vi "FindPrjLibItem.vi"(8 "error in (no error)":errorcluster, 10 "Item Name":string, 11 "Lib Path":path) -> (0 "error out":errorcluster, 3 "ProjectItem Refnum":refnum<vi>)   [LabVIEW 2020, in "CameraI2COUSB.lvlib" / "CameraDemo.lvclass"]
uses:
  CameraDemo.lvclass
  CameraDemo.lvclass/CameraDemo.ctl
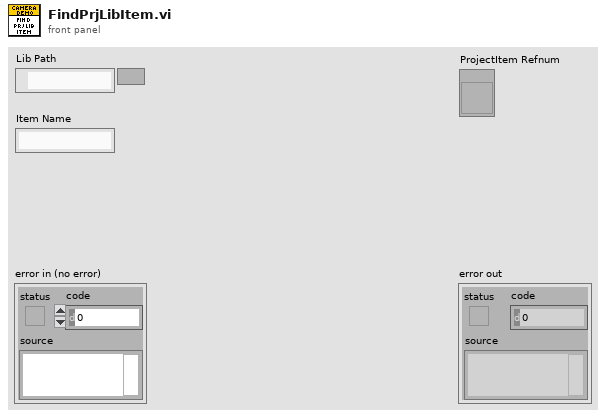
[diagram p1: front panel]
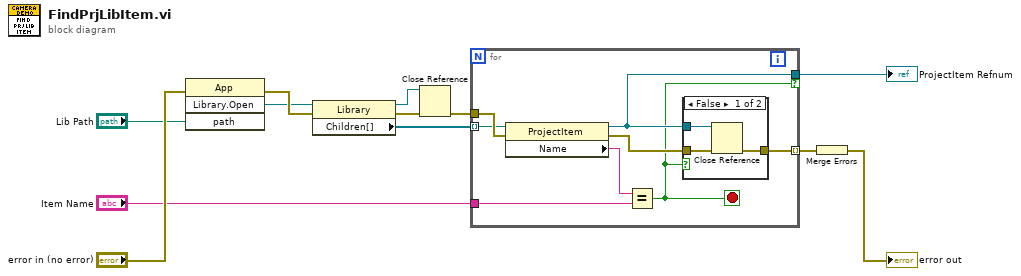
[diagram p0: block diagram]
diagram:
  n1 = invoke class="App" method="Library.Open"(error in="error in (no error)", "path"="Lib Path") -> (error out=w12:errorcluster, "Open Library"=w11:refnum<vi>)  [unwired: 2 in, 2 out]
  n2 = property class="Library"(reference=w11, error in=w12) -> (reference out=w9:refnum<vi>, error out=w10:errorcluster, "Children[]"=w7:refnum<vi>[])
  n3 = Close Reference(reference=w9, error in (no error)=w10) -> (error out=w8:errorcluster)
  n4 = for {
    tunnel: w7 -> [w16] mode=indexing
    tunnel: w8 -> [w19]
    tunnel: [w15] -> w3 mode=indexing
    tunnel: "Item Name" -> [w18]
    tunnel: [w14] -> w1 if=w13
    stop <- w13 stop-if-true
    n5 = property class="ProjectItem"(reference=w16, error in=w19) -> (reference out=w14:refnum<vi>, error out=w17:errorcluster, "Name"=w20:string)
    n6 = Equal?(x=w20, y=w18) -> (x = y?=w13:bool)
    n7 = case shown="False" w13 {
      tunnel: w17 -> [w23 w24]
      tunnel: w14 -> [w21 _]
      tunnel: [w22 w24] -> w15
      frame False {
        n8 = Close Reference(reference=w21, error in (no error)=w23) -> (error out=w22:errorcluster)
      }
      frame True {
      }
    }
  }
  "ProjectItem Refnum" <- w1
  n9 = Merge Errors(w3) -> (→"error out":errorcluster)
